vi "Train Tip SVM.vi"(8 "error in (no error)":errorcluster, 9 "Classifier File":path=path "C:/Users/Andrew/Documents/Apatite to Zircon Code/Track Finding/TipClassifier.knn", 10 "Non-tip Data File":path=path "C:/Users/Andrew/Documents/Apatite to Zircon Code/Track Finding/Non-tip Data.csv", 11 "Tip Data File":path=path "C:/Users/Andrew/Documents/Apatite to Zircon Code/Track Finding/Tip Data.csv") -> (0 "error out":errorcluster, 3 "Accuracy":sgl format="%.2f")   [LabVIEW 2013]
uses:
  <vilib>/vision/Classification.llb/IMAQ Classifier Nearest Neighbor options.ctl
  <vilib>/vision/Classification.llb/IMAQ SVM Kernel Options.ctl
  <vilib>/vision/Classification.llb/IMAQ SVM Model Options.ctl
  <vilib>/Utility/file.llb/Read From Spreadsheet File (DBL).vi
  <vilib>/vision/NI_Vision_Development_Module.lvlib
panel:
  out "Class Predictive Value":dbl[](array[numeric]) format="%.2f"
  out "Classification Distribution":i32[][](array[numeric])
  in  "Model Options":T1={"SVM Model"=enum."One Class", "Tolerance"=0.001, "Max. Iteration"=100000, "Nu"=0.1, "Shrinking"=TRUE, "Cost"=1.0, "Weighted Cost"=[]}
  in  "Kernel Options":T2={"Kernel"=enum."RBF", "Degree"=3, "Gamma"=1.0, "Coefficient"=0.0, "Sigma"=1.0, "Cache(MB)"=10.0}
  in  "Nearest Neighbor Options":T3={"Method"=1, "Metric"=2, "k"=4} {"Method" items=["Nearest Neighbor", "K Nearest Neighbor", "Minimum Mean Distance"]; "Metric" items=["Maximum", "Sum", "Euclidean"]; "k" min=3}
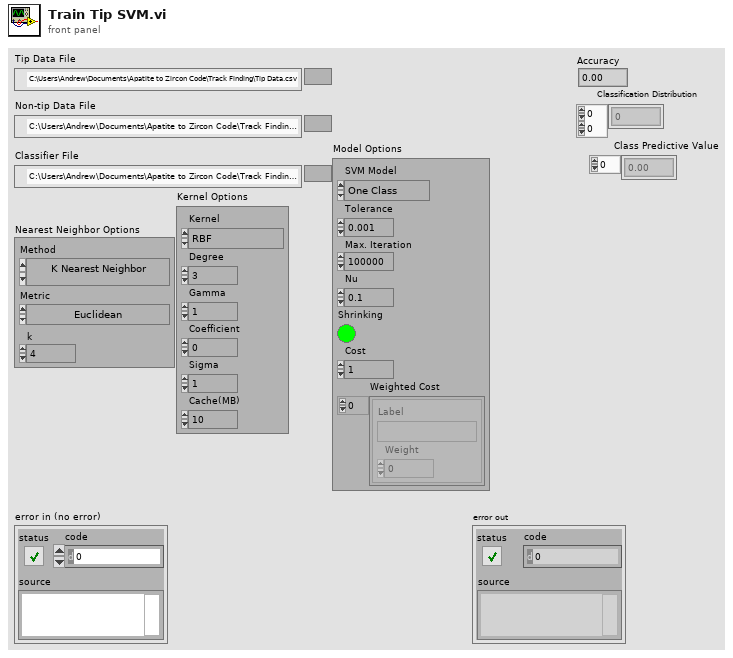
[diagram p1: front panel]
types:
  T1 = typedef "IMAQ SVM Model Options.ctl" = cluster{"SVM Model":enum32{"C-SVC", "nu-SVC", "One Class"}, "Tolerance":dbl, "Max. Iteration":i32, "Nu":dbl, "Shrinking":bool, "Cost":dbl, "Weighted Cost":cluster{"Label":string, "Weight":dbl}[]}
  T2 = typedef "IMAQ SVM Kernel Options.ctl" = cluster{"Kernel":enum32{"Linear", "Polynomial", "Gaussian", "RBF"}, "Degree":i32, "Gamma":dbl, "Coefficient":dbl, "Sigma":dbl, "Cache(MB)":dbl}
  T3 = typedef "IMAQ Classifier Nearest Neighbor options.ctl" = cluster{"Method":i32, "Metric":i32, "k":i32}
  T4 = typedef "Image Type" = u32
  T5 = typedef "IMAQ Image.ctl" = refnum<image>
  T6 = typedef "IMAQ Classifier Session.ctl" = refnum<k1>
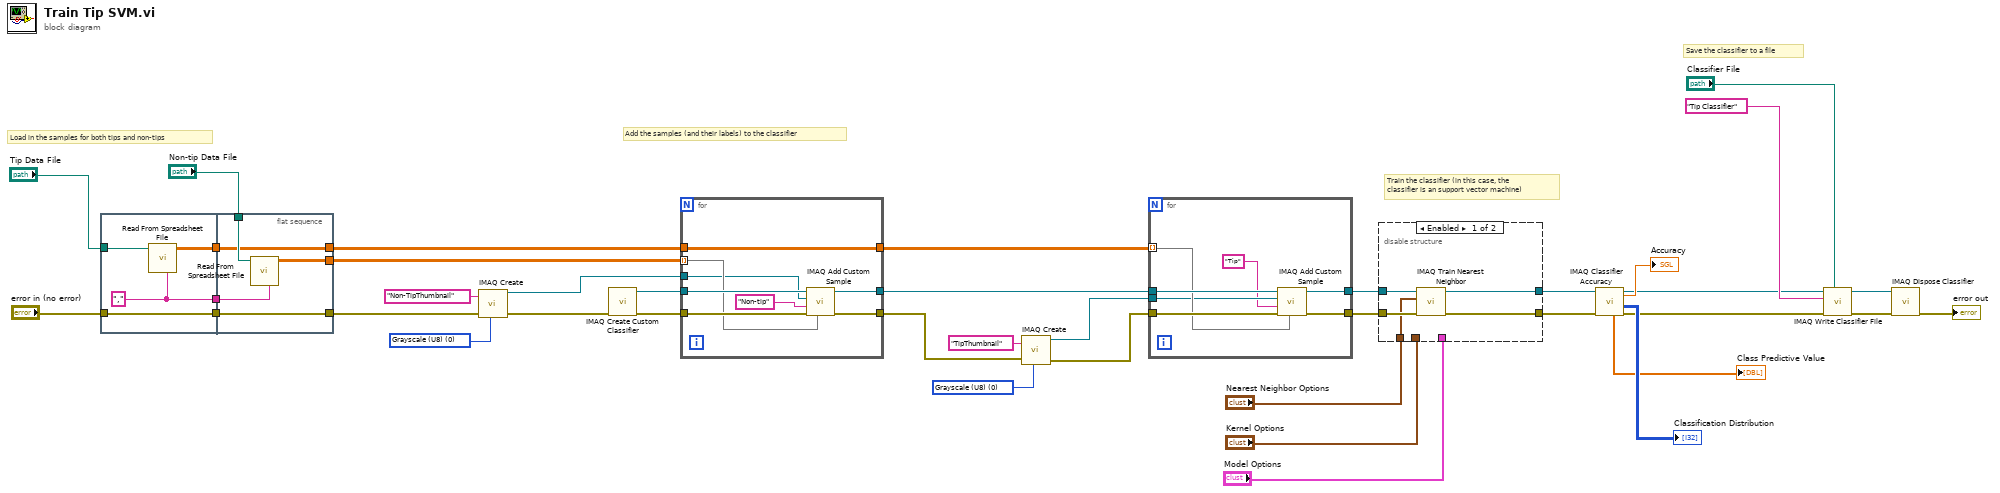
[diagram p0: block diagram]
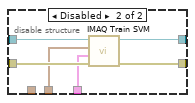
[diagram p2: hidden frame]
diagram:
  w28 = T4 0 items=["Grayscale (U8)", "Grayscale (I16)", "Grayscale (SGL)", "Complex (CSG)", "RGB (U32)", "HSL (U32)", "RGB (U64)", "Grayscale (U16)"] ("Image Type")
  w30 = T4 0 items=["Grayscale (U8)", "Grayscale (I16)", "Grayscale (SGL)", "Complex (CSG)", "RGB (U32)", "HSL (U32)", "RGB (U64)", "Grayscale (U16)"] ("Image Type")
  # "Save the classifier to a file"
  # "Train the classifier (in this case, the \nclassifier is an support vector machine)"
  # "Add the samples (and their labels) to the classifier"
  # "Load in the samples for both tips and non-tips"
  n1 = flat-sequence {
    tunnel: "Tip Data File" -> [w43]
    tunnel: "error in (no error)" -> [w42]
    tunnel: [w42] -> w37
    tunnel: [w41] -> w35
    tunnel: [w40] -> w23
    tunnel: [w48] -> w26
    tunnel: w37 -> [w48]
    tunnel: "Non-tip Data File" -> [w47]
    tunnel: [w46] -> w21
    tunnel: w35 -> [w45]
    tunnel: [w45] -> w22
    tunnel: w23 -> [w44]
    frame #0 {
      w40 = "," ("delimiter (\\t)")
      n2 = call-poly <vilib>:"Read From Spreadsheet File.vi"("delimiter (\\t)"=w40, "file path (dialog if empty)"=w43) -> ("all rows"=w41:dbl[][])  [unwired: 5 in, 4 out]
    }
    frame #1 {
      n3 = call-poly <vilib>:"Read From Spreadsheet File.vi"("delimiter (\\t)"=w44, "file path (dialog if empty)"=w47) -> ("all rows"=w46:dbl[][])  [unwired: 5 in, 4 out]
    }
  }
  n4 = call "IMAQ Create"("Image Name"="Non-TipThumbnail", "Image Type"=w28, "error in (no error)"=w26) -> ("New Image"=w20:T5, "error out"=w19:errorcluster)  [unwired: 2 in]
  n5 = call "IMAQ Create Custom Classifier"("error in (no error)"=w19) -> ("error out"=w33:errorcluster, "Classifier Session"=w34:T6)  [unwired: 9 in]
  n6 = for {
    tunnel: w21 -> [w54] mode=indexing
    tunnel: w34 -> [w55]
    tunnel: w33 -> [w56]
    tunnel: [w53] -> w31
    tunnel: [w52] -> w25
    tunnel: w22 -> [w51]
    tunnel: [w51] -> w32
    tunnel: w20 -> [w49]
    n7 = call "IMAQ Add Custom Sample"("Feature Vector"=w54, "error in (no error)"=w56, "Class"="Non-tip", "Image"=w49, "Classifier Session"=w55) -> ("error out"=w52:errorcluster, "Classifier Session (dup)"=w53:T6)  [unwired: 5 in]
  }
  n8 = call "IMAQ Create"("Image Name"="TipThumbnail", "Image Type"=w30, "error in (no error)"=w25) -> ("New Image"=w18:T5, "error out"=w17:errorcluster)  [unwired: 2 in]
  n9 = for {
    tunnel: w32 -> [w61] mode=indexing
    tunnel: w31 -> [w62]
    tunnel: w17 -> [w63]
    tunnel: [w60] -> w12
    tunnel: [w59] -> w11
    tunnel: w18 -> [w58]
    n10 = call "IMAQ Add Custom Sample"("Feature Vector"=w61, "error in (no error)"=w63, "Class"="Tip", "Image"=w58, "Classifier Session"=w62) -> ("error out"=w59:errorcluster, "Classifier Session (dup)"=w60:T6)  [unwired: 5 in]
  }
  n11 = disable-structure shown="Enabled" {
    disable-tunnel: w12 -> [w68 w74]
    disable-tunnel: w11 -> [w67 w73]
    disable-tunnel: "Nearest Neighbor Options" -> [w66 _]
    disable-tunnel: [w65 w70] -> w4
    disable-tunnel: [w64 w69] -> w3
    disable-tunnel: "Kernel Options" -> [_ w72]
    disable-tunnel: "Model Options" -> [_ w71]
    frame Enabled {
      n12 = call "IMAQ Train Nearest Neighbor"("error in (no error)"=w67, "Nearest Neighbor Options"=w66, "Classifier Session"=w68) -> ("error out"=w64:errorcluster, "Classifier Session (dup)"=w65:T6)  [unwired: 5 in, 2 out]
    }
    frame Disabled {
      n13 = call "IMAQ Train SVM"("error in (no error)"=w73, "Model Options"=w71, "Kernel Options"=w72, "Classifier Session"=w74) -> ("error out"=w69:errorcluster, "Classifier Session (dup)"=w70:T6)  [unwired: 4 in, 2 out]
    }
  }
  n14 = call "IMAQ Classifier Accuracy"("error in (no error)"=w3, "Classifier Session"=w4) -> ("error out"=w1:errorcluster, "Classification Distribution"=→"Classification Distribution":i32[][], "Classifier Session (dup)"=w2:T6, "Class Predictive Value"=→"Class Predictive Value":dbl[], "Accuracy"=→"Accuracy":sgl)  [unwired: 3 in, 2 out]
  n15 = call "IMAQ Write Classifier File"("File Path"="Classifier File", "error in (no error)"=w1, "Description"="Tip Classifier", "Classifier Session"=w2) -> ("error out"=w16:errorcluster, "Classifier Session (dup)"=w15:T6)  [unwired: 6 in]
  n16 = call "IMAQ Dispose Classifier"("error in (no error)"=w16, "Classifier Session"=w15) -> ("error out"=→"error out":errorcluster)  [unwired: 9 in]
